vi "Analyze Power Gain and SNR.vi"(7 "Published Data Id":string[](array[string]), 8 "error in (no error)":errorcluster, 9 "power spectrum":cluster{"f0":dbl, "df":dbl, "data":dbl[]}, 10 "power level (dBm)":dbl, 11 "Automation Refnum in":T1) -> (0 "error out":errorcluster, 1 "SNR (without harmonics)":dbl, 2 "Gain":dbl)   [LabVIEW 2014]
uses:
  <vilib>/NI_TestStand_SemiconductorModule/NI_TestStand_Semiconductor_Module.lvlibp/PinMap/General/SemiconductorModuleContext.ctl
  <vilib>/NI_TestStand_SemiconductorModule/NI_TestStand_Semiconductor_Module.lvlibp/PinMap/General/Publish/PublishDataDoubleFunctionalTest.vi
  <vilib>/NI_TestStand_SemiconductorModule/NI_TestStand_Semiconductor_Module.lvlibp
panel:
  out "Waveform Graph":cluster{"f0":dbl, "df":dbl, "data":dbl[]}(graph)
  out "detected fundamental\nfrequency [Hz]":dbl format="%.2f"
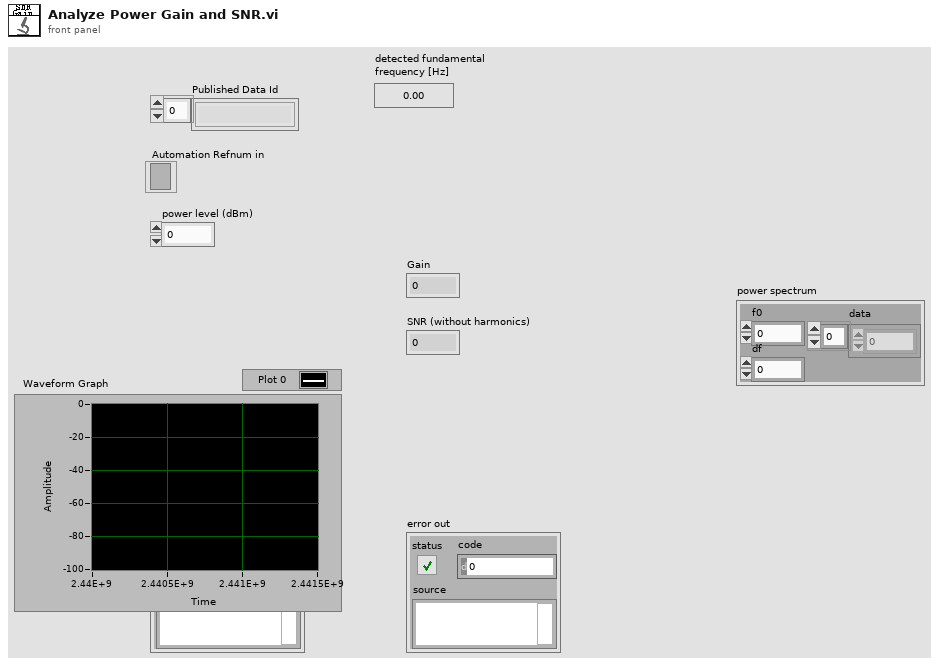
[diagram p1: front panel]
types:
  T1 = typedef "NI_TestStand_Semiconductor_Module.lvlibp/SemiconductorModuleContext.ctl" = refnum<k7>
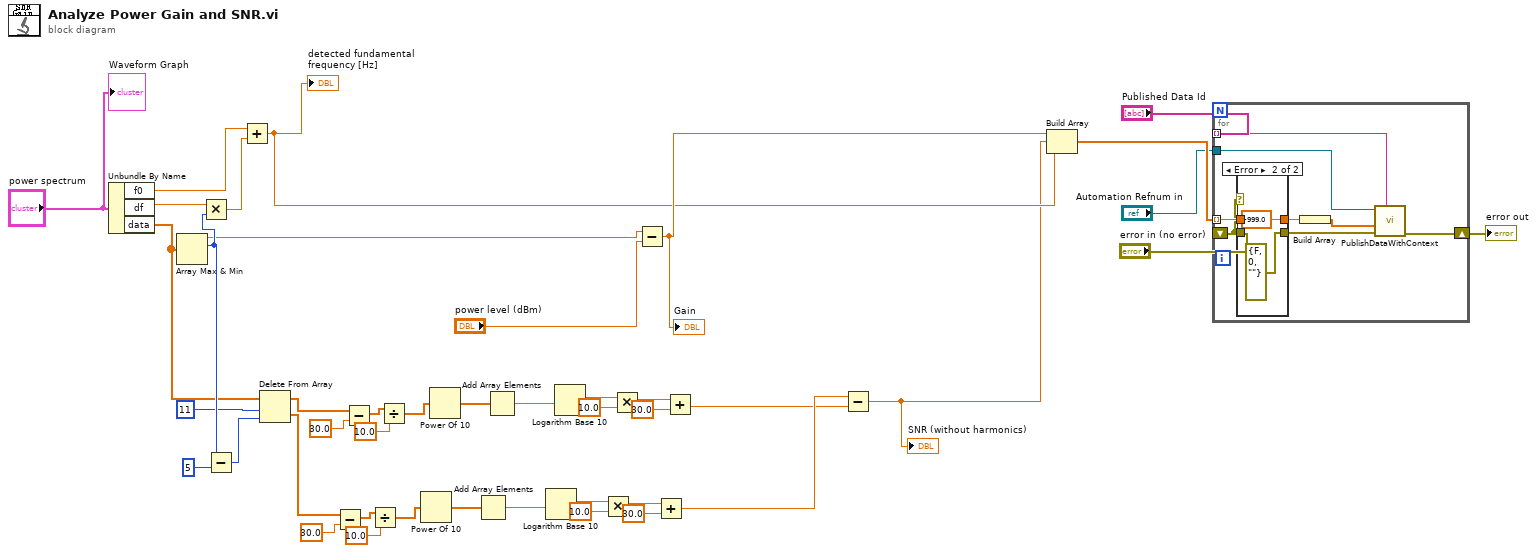
[diagram p0: block diagram]
diagram:
  n1 = Unbundle By Name("power spectrum") -> ("f0"=w23:dbl, "df"=w22:dbl, "data"=w1:dbl[])
  n2 = Array Max & Min(array=w1) -> (max value=w2:dbl, max index (indices)=w21:i32)  [unwired: 2 out]
  n3 = Multiply(x=w22, y=w21) -> (x*y=w20:dbl)
  n4 = Subtract(x=w21, y=5) -> (x-y=w18:i32)
  n5 = Add(x=w23, y=w20) -> (x+y=w19:dbl)
  "detected fundamental\nfrequency [Hz]" <- w19
  n6 = Delete From Array(array=w1, length=11, index=w18) -> (deleted portion=w3:dbl[], array with subset deleted=w7:dbl[])
  n7 = Subtract(x=w3, y=30.0) -> (x-y=w33:dbl[])
  n8 = Subtract(x=w7, y=30.0) -> (x-y=w15:dbl[])
  n9 = Divide(x=w33, y=10.0) -> (x/y=w34:dbl[])
  n10 = Divide(x=w15, y=10.0) -> (x/y=w16:dbl[])
  n11 = Power Of 10(x=w34) -> (10^x=w31:dbl[])
  n12 = Power Of 10(x=w16) -> (10^x=w13:dbl[])
  n13 = Add Array Elements(numeric array=w31) -> (sum=w30:dbl)
  n14 = Add Array Elements(numeric array=w13) -> (sum=w12:dbl)
  n15 = Logarithm Base 10(1:w30) -> (0:w29:dbl)
  n16 = Logarithm Base 10(1:w12) -> (0:w11:dbl)
  n17 = Multiply(x=w29, y=10.0) -> (x*y=w27:dbl)
  n18 = Multiply(x=w11, y=10.0) -> (x*y=w9:dbl)
  n19 = Subtract(x=w2, y="power level (dBm)") -> (x-y=w41:dbl)
  "Gain" <- w41
  n20 = Add(x=w27, y=30.0) -> (x+y=w24:dbl)
  n21 = Add(x=w9, y=30.0) -> (x+y=w6:dbl)
  n22 = Subtract(x=w24, y=w6) -> (x-y=w5:dbl)
  "SNR (without harmonics)" <- w5
  n23 = Build Array(w41, w5, w19) -> (w42:dbl[])
  n24 = for {
    tunnel: "Automation Refnum in" -> [w50]
    tunnel: "Published Data Id" -> [w49] mode=indexing
    shift-right: [w51] -> w39
    shift-left: "error in (no error)" -> [w45]
    tunnel: w42 -> [w47] mode=indexing
    n25 = case shown="Error" w45 {
      tunnel: w47 -> [w53 _]
      tunnel: [w53 -999.0] -> w46
      tunnel: w45 -> [w52 _]
      tunnel: [w52 errorcluster {"status"=FALSE, "code"=0, "source"=""} ("error constant")] -> w44
      frame No Error {
      }
      frame Error {
      }
    }
    n26 = Build Array(w46) -> (w48:dbl[])
    n27 = call-poly <vilib>:"PublishDataWithContext.vi"("Published Data Id"=w49, "error in (no error)"=w44, "Data In"=w48, "Semiconductor Module Context"=w50) -> ("error out"=w51:errorcluster)  [unwired: 6 in, 1 out]
  }
  "error out" <- w39
  "Waveform Graph" <- "power spectrum"
